vi "Auto Update SketchBody Number.vi"(10 "Sketch # in":i32, 11 "Feature In":string) -> (2 "resulting string":string, 3 "Sketch # out":i32)   [LabVIEW 2019]
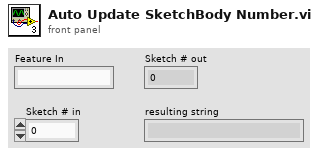
[diagram p1: front panel]
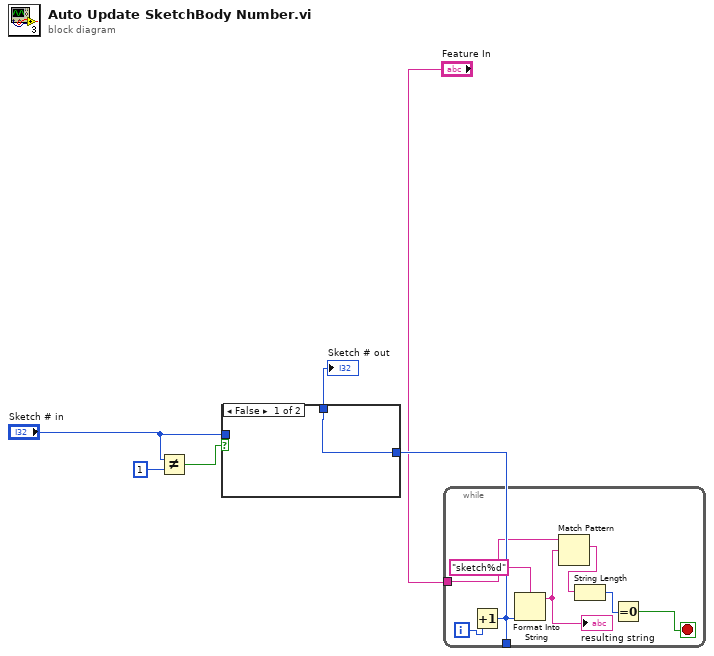
[diagram p0: block diagram]
diagram:
  n1 = Not Equal?(x="Sketch # in", y=1) -> (x != y?=w3:bool)
  n2 = while {
    tunnel: "Feature In" -> [w14]
    tunnel: [w7] -> w6
    i -> [w12]
    stop <- w8 stop-if-true
    n3 = Increment(x=w12) -> (x+1=w7:i32)
    n4 = Format Into String(format string="sketch%d", w7) -> (resulting string=w11:string)  [unwired: 2 in, 1 out]
    "resulting string" <- w11
    n5 = Match Pattern(string=w14, regular expression=w11) -> (match substring=w10:string)  [unwired: 1 in, 3 out]
    n6 = String Length(string=w10) -> (length=w9:i32)
    n7 = Equal To 0?(x=w9) -> (x = 0?=w8:bool)
  }
  n8 = case shown="False" w3 {
    tunnel: [w15 w16] -> w4
    tunnel: "Sketch # in" -> [_ w16]
    tunnel: w6 -> [w15 _]
    frame False {
    }
    frame True {
    }
  }
  "Sketch # out" <- w4
